vi "Get or Create Command.vi"(8 "error in (no error)":errorcluster, 11 "Message Refnum In":T1 format="%.0x") -> (0 "error out":errorcluster, 2 "Command Refnum":T1 format="%.0x", 3 "Message Refnum Out":T1 format="%.0x")   [LabVIEW 2018, in "Instrument Addon Scripting API.lvlib"]
uses:
  Instrument Addon Scripting API.lvlib
  <vilib>/NI Veristand/Custom Device API/Custom Device Item Ref.ctl
  Addon/Addon Shared/SubVIs/Constants.vi
  <vilib>/NI Veristand/Custom Device Tools/Custom Device Utility Library/NI VeriStand - Search for Item by GUID.vi
  <vilib>/NI Veristand/Custom Device Tools/Custom Device Utility Library/Custom Device Utility Library.lvlib
  Addon/Addon Shared/Instrument Addon Shared.lvlib
  <vilib>/NI Veristand/Custom Device API/Custom Device API.lvlib
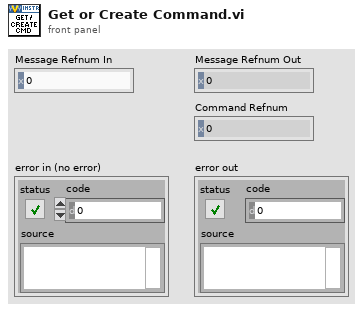
[diagram p1: front panel]
types:
  T1 = typedef "Custom Device API.lvlib/Custom Device Item Ref.ctl" = u64
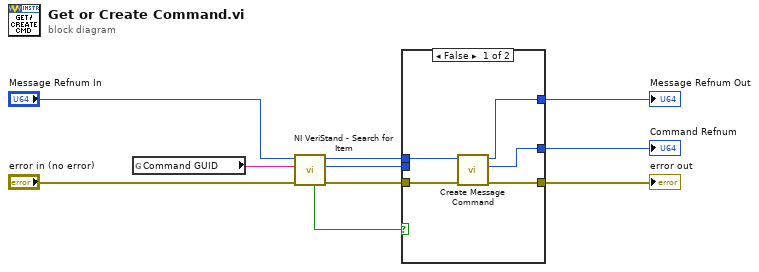
[diagram p0: block diagram]
diagram:
  n1 = global read "Constants.vi" "Command GUID"() -> (w10:string)
  n2 = call-poly <vilib>:"NI VeriStand - Search for Item.vi"("error in"="error in (no error)", "Item GUID"=w10, "Section Ref in"="Message Refnum In") -> ("error out"=w4:errorcluster, "Item Ref"=w5:T1, "Section Ref out"=w6:T1, "Found"=w7:bool)  [unwired: 5 in]
  n3 = case shown="False" w7 {
    tunnel: w6 -> [w13 w18]
    tunnel: w5 -> [_ w17]
    tunnel: w4 -> [w15 w16]
    tunnel: [w12 w18] -> w3
    tunnel: [w11 w17] -> w2
    tunnel: [w14 w16] -> w1
    frame False {
      n4 = call "Create Message Command.vi"("error in (no error)"=w15, "Message in"=w13) -> ("error out"=w14:errorcluster, "Command out"=w11:T1, "Message out"=w12:T1)  [unwired: 7 in]
    }
    frame True {
    }
  }
  "Message Refnum Out" <- w3
  "error out" <- w1
  "Command Refnum" <- w2
